vi "日志信息主动发送(子VI).vi"   [LabVIEW 2016, in "数据传输系统-03.lvlib"]
types:
  T1 = typedef "LVDateTimeRec.ctl" = cluster{"秒数的小数部分":dbl, "秒":i32, "分":i32, "时":i32, "日":i32, "月":i32, "年":i32, "天数（周）":i32, "天数（年）":i32, "DST":i32}
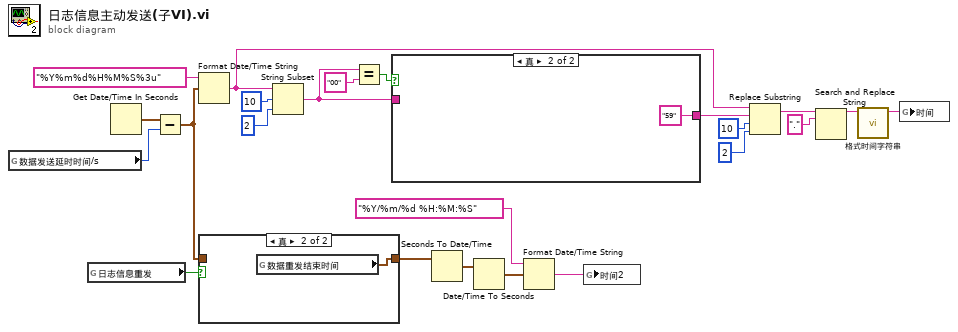
[diagram p0: block diagram]
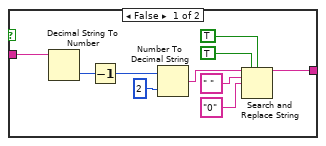
[diagram p3: hidden frame]
diagram:
  n1 = global read "断电保存全局.vi" "数据发送延时时间/s"() -> (w8:i32)
  n2 = global read "断电保存全局.vi" "日志信息重发"() -> (w3:bool)
  n3 = Get Date/Time In Seconds() -> (seconds since 1Jan1904=w7:timestamp)
  n4 = Subtract(x=w7, y=w8) -> (x-y=w2:timestamp)
  n5 = Format Date/Time String(time format string (%c)="%Y%m%d%H%M%S%3u" ("时间格式字符串(%c)"), seconds (now)=w2) -> (date/time string=w12:string)  [unwired: 1 in]
  n6 = case shown="真" w3 {
    tunnel: w2 -> [w24 _]
    tunnel: [w24 w25] -> w1
    frame False {
    }
    frame True {
      n7 = global read "断电保存全局.vi" "数据重发结束时间"() -> (w25:timestamp)
    }
  }
  n8 = String Subset(string=w12, offset (0)=10 ("偏移量(0)"), length (rest)=2 ("长度（子字符串长度）")) -> (substring=w20:string)
  n9 = Equal?(x=w20, y="00") -> (x = y?=w19:bool)
  n10 = case shown="真" w19 {
    tunnel: w20 -> [w35 _]
    tunnel: [w27 "59" ("y")] -> w21
    frame False {
      n11 = Decimal String To Number(string=w35) -> (number=w34:i32)  [unwired: 2 in, 1 out]
      n12 = Decrement(x=w34) -> (x-1=w28:i32)
      n13 = Number To Decimal String(number=w28, width (-)=i16 2 ("宽度(-)")) -> (decimal integer string=w30:string)
      n14 = Search and Replace String(replace all?=TRUE ("替换全部？(F)"), case sensitive?=TRUE ("忽略大小写？(F)"), input string=w30, search string=" " ("搜索字符串"), replace string="0" ("替换字符串(\"\")")) -> (result string=w27:string)  [unwired: 3 in, 3 out]
    }
    frame True {
    }
  }
  n15 = Seconds To Date/Time(time stamp (now)=w1) -> (date time rec=w4:T1)  [unwired: 1 in]
  n16 = Date/Time To Seconds(2:w4) -> (0:w6:timestamp)  [unwired: 1 in]
  n17 = Format Date/Time String(time format string (%c)="%Y/%m/%d %H:%M:%S" ("时间格式字符串(%c)"), seconds (now)=w6) -> (date/time string=w11:string)  [unwired: 1 in]
  n18 = global write "全局 时间2.vi" "时间2"(w11) -> ()
  n19 = Replace Substring(2:2 ("长度（子字符串长度）"), 3:10 ("偏移量(0)"), 4:w21, 5:w12) -> (1:w13:string)  [unwired: 1 out]
  n20 = Search and Replace String(input string=w13, search string="." ("搜索字符串")) -> (result string=w9:string)  [unwired: 6 in, 3 out]
  n21 = call "格式时间字符串.vi"("字符串"=w9) -> ("连接的字符串"=w14:string)  [unwired: 10 in]
  n22 = global write "全局 水样时间.vi" "时间"(w14) -> ()
